vi "Graph_3_Signal.vi"(8 "y":timestamp, 9 "Dynamic Data 3":dbl, 10 "Dynamic Data Type 2":dbl, 11 "Dynamic Data Type":dbl) -> (3 "Signals":dynamicdata(graph))   [LabVIEW 2019]
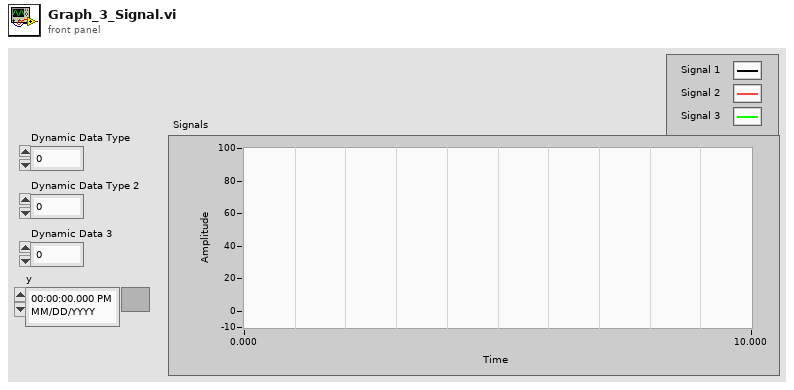
[diagram p1: front panel]
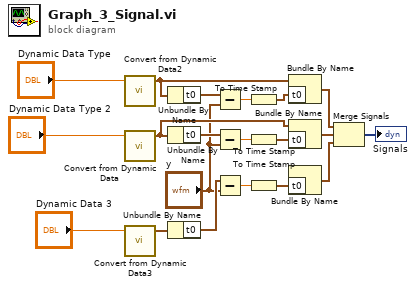
[diagram p0: block diagram]
diagram:
  n1 = call "Convert from Dynamic Data2"("Dynamic Data Type"="Dynamic Data Type") -> ("Waveform"=w15:waveform(dbl))  [unwired: 3 in]
  n2 = call "Convert from Dynamic Data"("Dynamic Data Type"="Dynamic Data Type 2") -> ("Waveform"=w20:waveform(dbl))  [unwired: 3 in]
  n3 = call "Convert from Dynamic Data3"("Dynamic Data Type"="Dynamic Data 3") -> ("Waveform"=w9:waveform(dbl))  [unwired: 3 in]
  n4 = Unbundle By Name ("Get Waveform Components 2")(w15) -> ("t0"=w12:timestamp)
  n5 = Unbundle By Name ("Get Waveform Components")(w20) -> ("t0"=w16:timestamp)
  n6 = Unbundle By Name ("Get Waveform Components 3")(w9) -> ("t0"=w6:timestamp)
  n7 = Subtract ("Subtract 2")(x=w12, y="y") -> (x-y=w14:dbl)
  n8 = Subtract(x=w16, y="y") -> (x-y=w19:dbl)
  n9 = Subtract ("Subtract 3")(x=w6, y="y") -> (x-y=w8:dbl)
  n10 = To Time Stamp ("To Time Stamp 2")(1:w14) -> (0:w13:timestamp)
  n11 = To Time Stamp(1:w19) -> (0:w18:timestamp)
  n12 = To Time Stamp ("To Time Stamp 3")(1:w8) -> (0:w7:timestamp)
  n13 = Bundle By Name ("Build Waveform 2")(cluster=w15, "t0"=w13) -> (w11:waveform(dbl))
  n14 = Bundle By Name ("Build Waveform")(cluster=w20, "t0"=w18) -> (w17:waveform(dbl))
  n15 = Bundle By Name ("Build Waveform 3")("t0"=w7) -> (w3:waveform(dbl))  [unwired: 1 in]
  n16 = Merge Signals(w11, w17, w3) -> (→"Signals":dynamicdata)
